vi "Sensor_Force.vi"() -> ()   [LabVIEW 2018]
panel:
  out "Force(N)":dbl[](array[numeric])
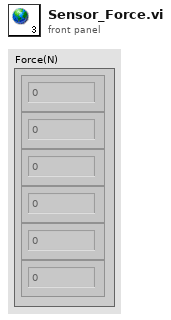
[diagram p1: front panel]
diagram:
